vi "NI.InterfaceBD_Test.vi"() -> ()   [LabVIEW 2012, in "Lib_UEL.ATE.lvlib" / "Lib_PCI6221.lvlib"]
uses:
  Lib_PCI6221.lvlib
panel:
  out "剩余元素":string[](array[string])
  out "TestLog":string
  out "error out":errorcluster caption="Error Out"
  in  "DAQmx Device":tag
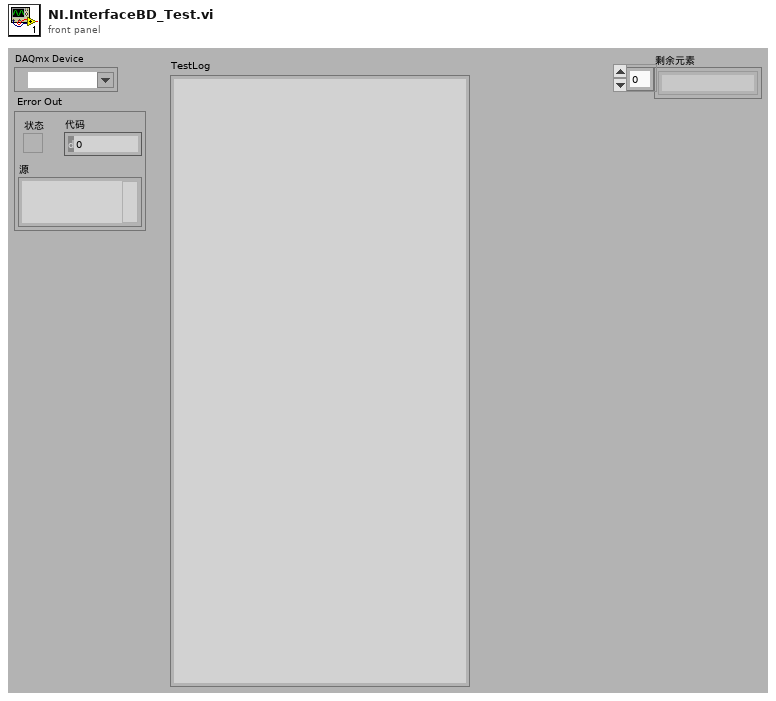
[diagram p1: front panel]
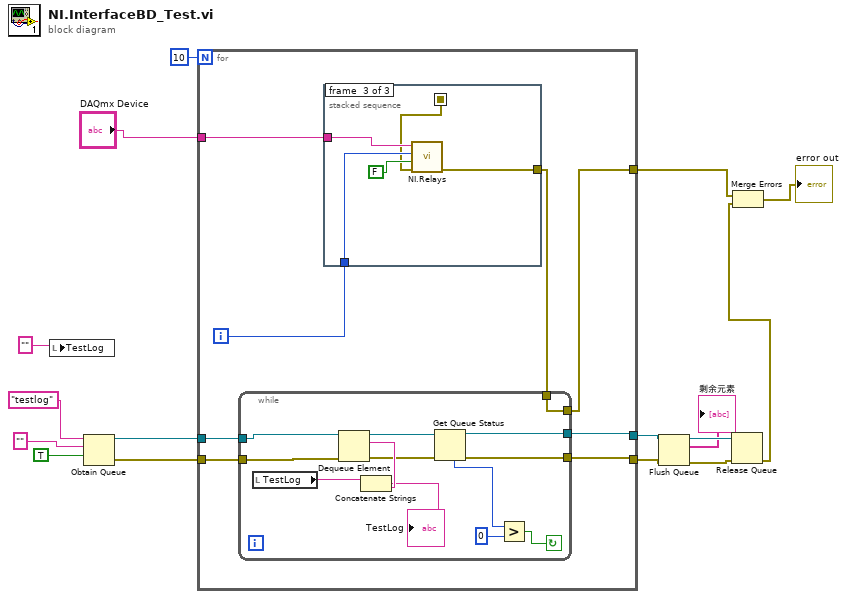
[diagram p0: block diagram]
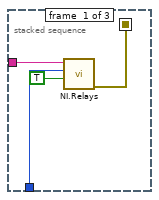
[diagram p2: hidden frame]
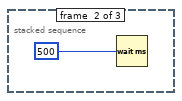
[diagram p3: hidden frame]
diagram:
  n1 = local write "TestLog"("" ("TestLog")) -> ()
  n2 = Obtain Queue(name (unnamed)="testlog" ("名称（未命名）"), element data type="" ("名称（未命名）"), create if not found? (T)=TRUE ("如未找到是否创建？(T)")) -> (queue out=w5:refnum<queue>, error out=w4:errorcluster)  [unwired: 2 in, 1 out]
  n3 = for {
    N: 10 -> [_]
    tunnel: [w17] -> w10
    tunnel: "DAQmx Device" -> [w24]
    tunnel: w5 -> [w22]
    tunnel: w4 -> [w21]
    tunnel: [w19] -> w3
    tunnel: [w20] -> w2
    i -> [w23]
    n4 = stacked-sequence {
      seq-local: [w38 _ _] -> [_ _ w44]
      tunnel: w24 -> [w41 _ w47]
      tunnel: w23 -> [w40 _ w46]
      tunnel: [_ _ w43] -> w18
      frame #0 {
        n5 = call "NI.Relays.vi"("Relay.ON.OFF"=TRUE, "Relay"=w40, "DAQmx Device"=w41) -> ("error out"=w38:errorcluster)  [unwired: 8 in]
      }
      frame #1 {
        n6 = Wait (ms)(milliseconds to wait=u32 500 ("等待时间（毫秒）")) -> ()  [unwired: 1 out]
      }
      frame #2 {
        n7 = call "NI.Relays.vi"("error in"=w44, "Relay.ON.OFF"=FALSE, "Relay"=w46, "DAQmx Device"=w47) -> ("error out"=w43:errorcluster)  [unwired: 7 in]
      }
    }
    n8 = while {
      tunnel: w22 -> [w34]
      tunnel: w21 -> [w33]
      tunnel: [w30] -> w20
      tunnel: [w29] -> w19
      tunnel: [w25] -> w17
      tunnel: w18 -> [w25]
      stop <- w26 continue-if-true
      n9 = local read "TestLog"() -> (w36:string)
      n10 = Dequeue Element(queue=w34, error in (no error)=w33) -> (queue out=w32:refnum<queue>, element=w37:string, error out=w31:errorcluster)  [unwired: 1 in, 1 out]
      n11 = Concatenate Strings(w36, w37) -> (→"TestLog":string)
      n12 = Get Queue Status(queue=w32, error in (no error)=w31) -> (queue out=w29:refnum<queue>, error out=w30:errorcluster, # elements in queue=w28:i32)  [unwired: 1 in, 5 out]
      n13 = Greater?(x=w28, y=0) -> (0:w26:bool)
    }
  }
  n14 = Flush Queue(queue=w3, error in (no error)=w2) -> (queue out=w14:refnum<queue>, remaining elements=→"剩余元素":string[], error out=w13:errorcluster)
  n15 = Release Queue(queue=w14, error in (no error)=w13) -> (error out=w11:errorcluster)  [unwired: 1 in, 2 out]
  n16 = Merge Errors(w10, w11) -> (→"error out":errorcluster)
